vi "Main.vi"() -> ()   [LabVIEW 2017]
doc: "The myRIO Project template acquires acceleration data from the onboard accelerometer and displays the changes of acceleration values in a waveform chart."
uses:
  <vilib>/myRIO/Instrument Drivers/Utilities/Utilities.lvlib
panel:
  out "Relación":dbl
  in  "Calibrar":bool
  in  "Home":bool
  in  "Ir_posicion":bool
  in  "Fijar Posición":dbl
  out "Posición en X":dbl
  in  "Abajo_X":bool
  in  "Arriba_X":bool
  in  "Avance":dbl
  out "error out":errorcluster
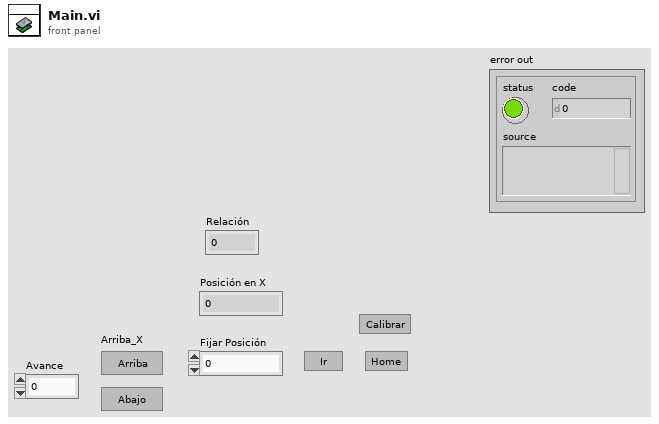
[diagram p1: front panel]
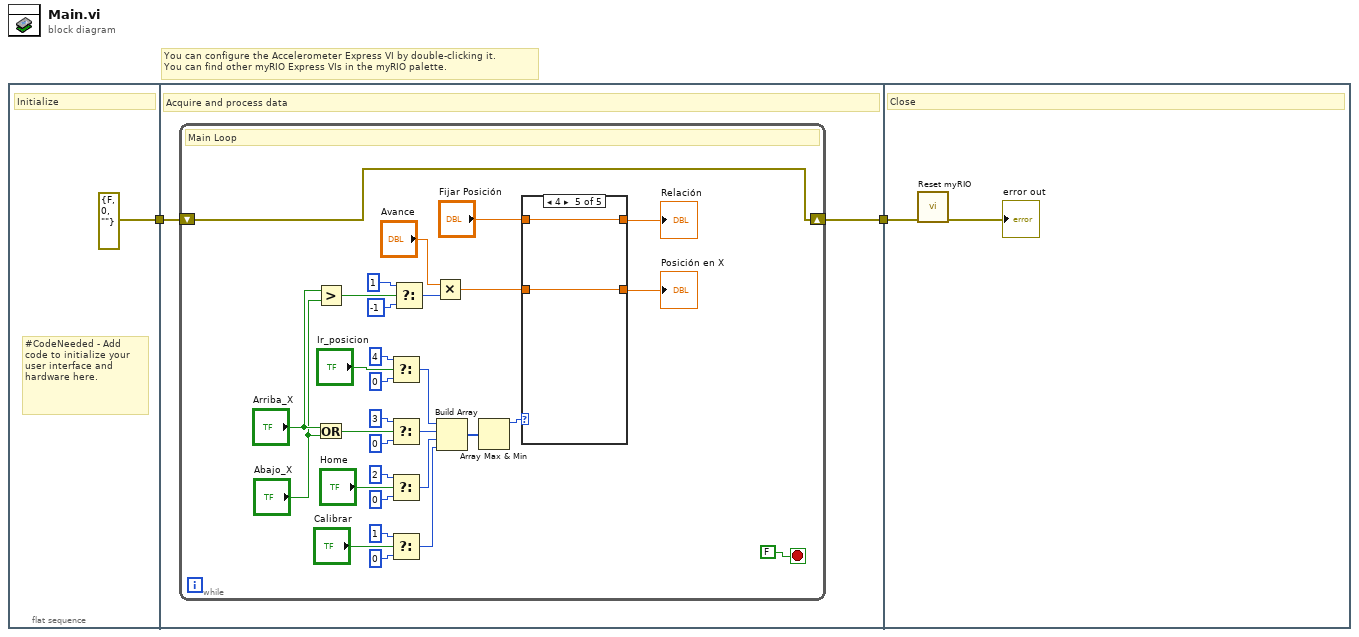
[diagram p0: block diagram]
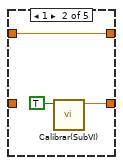
[diagram p3: hidden frame]
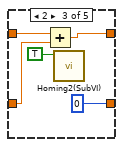
[diagram p4: hidden frame]
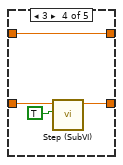
[diagram p5: hidden frame]
diagram:
  # "You can configure the Accelerometer Express VI by double-clicking it.\nYou can find other myRIO Express VIs in the myRIO palette."
  n1 = flat-sequence {
    tunnel: [errorcluster {"status"=FALSE, "code"=0, "source"=""} ("error in (no error)")] -> w2
    tunnel: w2 -> [w5]
    tunnel: [w4] -> w1
    tunnel: w1 -> [w54]
    frame #0 {
      # "#CodeNeeded - Add code to initialize your user interface and hardware here."
      # "Initialize"
    }
    frame #1 {
      # "Acquire and process data"
      n2 = while {
        shift-right: [w7] -> w4
        shift-left: w5 -> [w7]
        stop <- FALSE stop-if-true
        # "Main Loop"
        n3 = Greater?(x="Arriba_X", y="Abajo_X") -> (0:w15:bool)
        n4 = Or(x="Arriba_X", y="Abajo_X") -> (x .or. y?=w26:bool)
        n5 = Select(t=4, s="Ir_posicion", f=0) -> (s? t:f=w24:i32)
        n6 = Select(t=3, s=w26, f=0) -> (s? t:f=w23:i32)
        n7 = Select(t=2, s="Home", f=0) -> (s? t:f=w22:i32)
        n8 = Select(t=1, s="Calibrar", f=0) -> (s? t:f=w21:i32)
        n9 = Select(t=1, s=w15, f=-1) -> (s? t:f=w11:i32)
        n10 = Multiply(x="Avance", y=w11) -> (x*y=w10:dbl)
        n11 = Build Array(w24, w23, w22, w21) -> (w20:i32[])
        n12 = Array Max & Min(array=w20) -> (max value=w19:i32)  [unwired: 3 out]
        n13 = case shown="4" w19 {
          tunnel: [w37 w40 0 w48 w52] -> w18
          tunnel: w10 -> [w37 _ w44 w50 w52]
          tunnel: [w38 w39 w42 w47 w51] -> w9
          tunnel: "Fijar Posición" -> [w38 w39 w43 w47 w51]
          frame 0, Default {
          }
          frame 1 {
            n14 = call "Calibrar(SubVI).vi"("Calibrar"=TRUE) -> ("Relación"=w40:dbl)  [unwired: 10 in]
          }
          frame 2 {
            n15 = Add(x=w43, y=w44) -> (x+y=w42:dbl)
            n16 = call "Homing2(SubVI).vi"("Home"=TRUE) -> ()  [unwired: 10 in, 1 out]
          }
          frame 3 {
            n17 = call "Step (SubVI).vi"("Mover"=TRUE, "Step"=w50) -> ("Numeric"=w48:dbl)  [unwired: 9 in]
          }
          frame 4 {
          }
        }
        "Posición en X" <- w18
        "Relación" <- w9
      }
    }
    frame #2 {
      # "Close"
      n18 = call <vilib>:"Reset myRIO.vi"("error in (no error)"=w54) -> ("error out"=→"error out":errorcluster)  [unwired: 10 in]
    }
  }
